vi "Read uL_ms.vi"(8 "error in (no error)":errorcluster, 11 "TTLWaterDelivery in":refnum<class "TTLWaterDelivery.lvclass">) -> (0 "error out":errorcluster, 2 "uL/ms":dbl, 3 "TTLWaterDelivery out":refnum<class "TTLWaterDelivery.lvclass">)   [LabVIEW 2020, in "TTLWaterDelivery.lvclass"]
uses:
  TTLWaterDelivery.lvclass
  TTLWaterDelivery.lvclass/TTLWaterDelivery.ctl
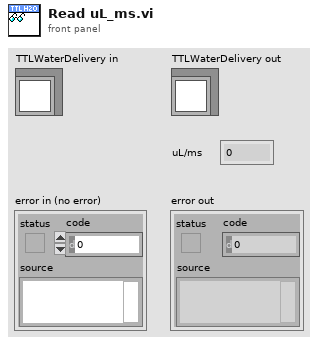
[diagram p1: front panel]
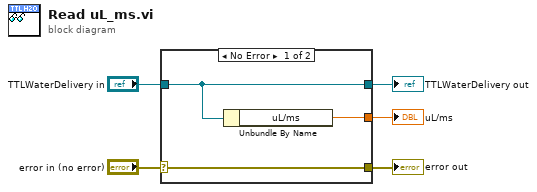
[diagram p0: block diagram]
diagram:
  n1 = case shown="No Error" "error in (no error)" {
    selector: "error in (no error)" -> [w8 w9]
    tunnel: [w8 w9] -> w4
    tunnel: [w7 w10] -> w2
    tunnel: "TTLWaterDelivery in" -> [w7 w10]
    tunnel: [w6 _] -> w1
    frame No Error {
      n2 = Unbundle By Name(w7) -> ("uL/ms"=w6:dbl)
    }
    frame Error {
    }
  }
  "error out" <- w4
  "TTLWaterDelivery out" <- w2
  "uL/ms" <- w1
